vi "Vicon2JointAngles.vi"(5 "Thigh Reference (to Hip)":enum16{"Hip", "Ground"}(ring), 6 "Operation(GetData)":T1, 7 "JointAngleDir([-1,1,1,-1])":dbl[](array[numeric])=[-1.0, 1.0, 1.0, -1.0], 8 "error in (no error)":errorcluster, 9 "LockHipAbduction(F)":bool, 10 "LockHipRotation(T)":bool=TRUE, 11 "ViconIMU in (rad)":dbl[](array[numeric])) -> (0 "error out":errorcluster, 3 "Joint Angles (rad)":dbl[](array[numeric]) format="%#.4f")   [LabVIEW 2016]
uses:
  <vilib>/Analysis/Matrix/Datatypes/RealMatrix.ctl
  HighLevelController/TypeDef/IMU_operation.ctl
  <vilib>/Analysis/coordinate.llb/Euler Rotation Order.ctl
  <vilib>/Analysis/BLAS.llb/LV_Transpose.ctl
  Classes/SerialChain/TypeDef/xyzO.ctl
  <vilib>/Analysis/Matrix/Numeric/Conversions/Array To Matrix - RA2.vi
  <vilib>/Analysis/BLAS.llb/dgemm - General Matrix-Matrix Product (DBL).vi
  <vilib>/Analysis/7linalg.llb/Create Special Real Matrix.vi
  <vilib>/Analysis/NI_AALPro.lvlib
  <vilib>/Analysis/NI_AALBLAS.lvlib
  <vilib>/Analysis/Matrix/NI_Matrix.lvlib
  Classes/SerialChain/SerialChain.lvclass
panel:
  out "R_CtoS_Shank":T2 format="%#.3f"
  out "R_CtoS_Thigh":T2 format="%#.3f"
  out "R_CtoS_Hip":T2 format="%#.3f"
  out "R0":T2 format="%#.3f"
  in  "UseStandPos(T)":bool=TRUE
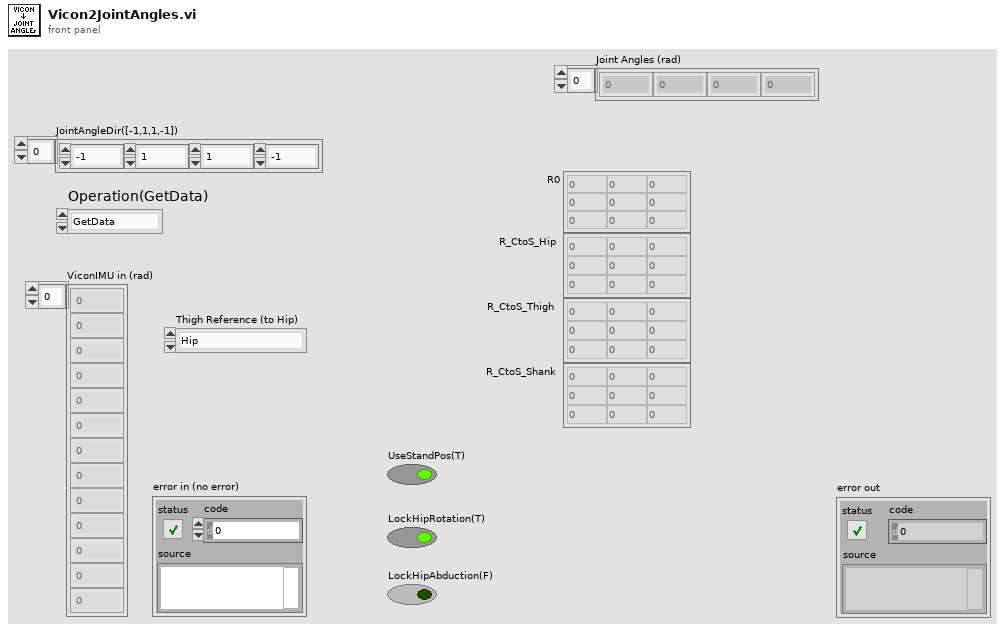
[diagram p1: front panel]
types:
  T1 = typedef "IMU_operation.ctl" = enum16{"GetData", "ClearStandPos", "SetStandPos"}
  T2 = typedef "NI_Matrix.lvlib/RealMatrix.ctl" = dbl[][]
  T3 = typedef "SerialChain.lvclass/xyzO.ctl" = enum16{"X", "Y", "Z", "O"}
  T4 = typedef "NI_AALPro.lvlib/Euler Rotation Order.ctl" = u16
  T5 = typedef "NI_AALBLAS.lvlib/LV_Transpose.ctl" = i32
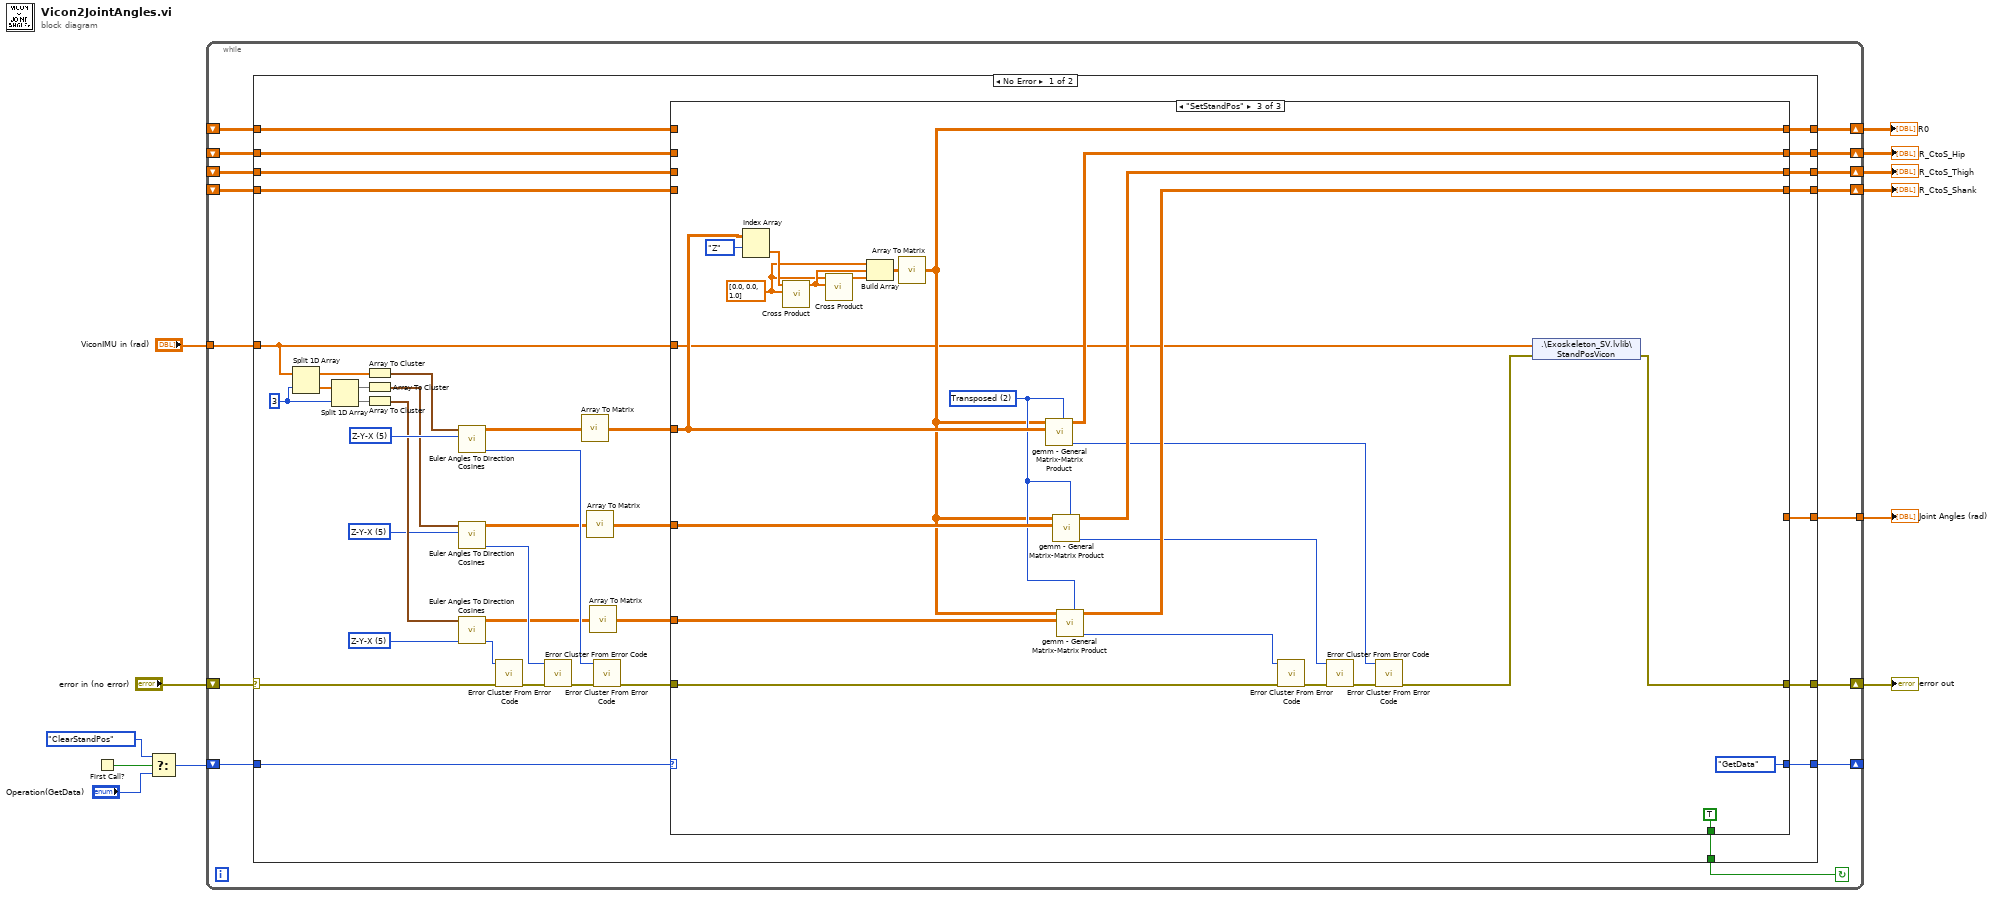
[diagram p0: block diagram]
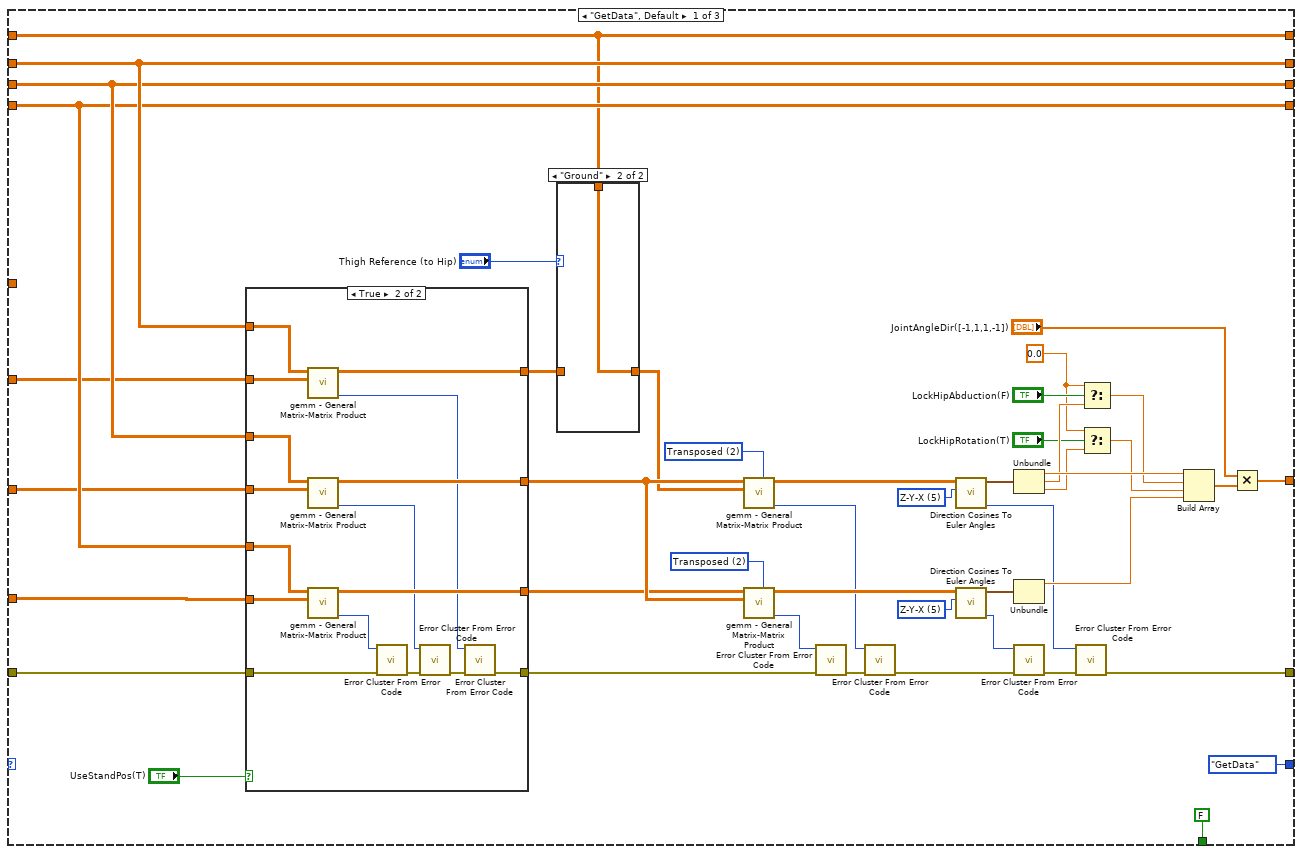
[diagram p2: hidden frame]
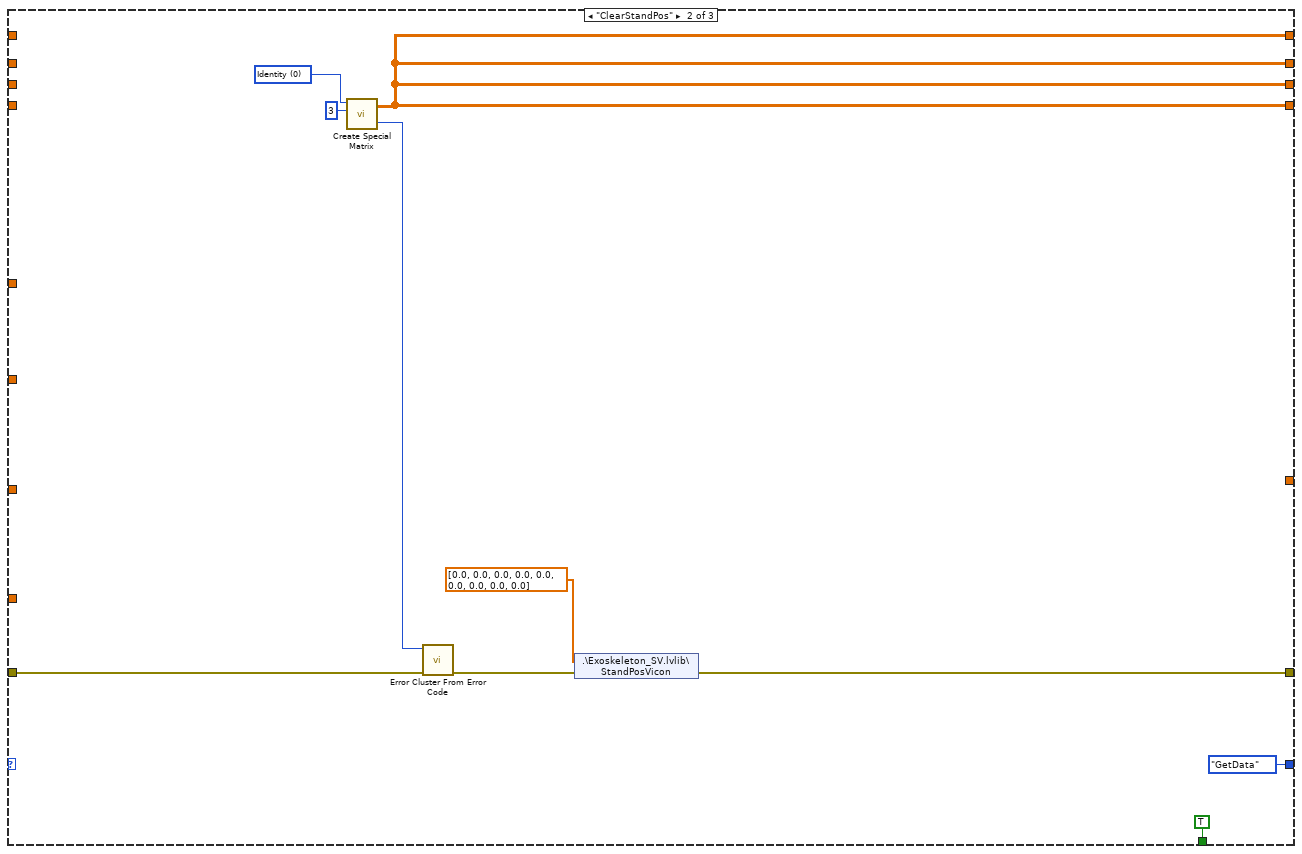
[diagram p5: hidden frame]
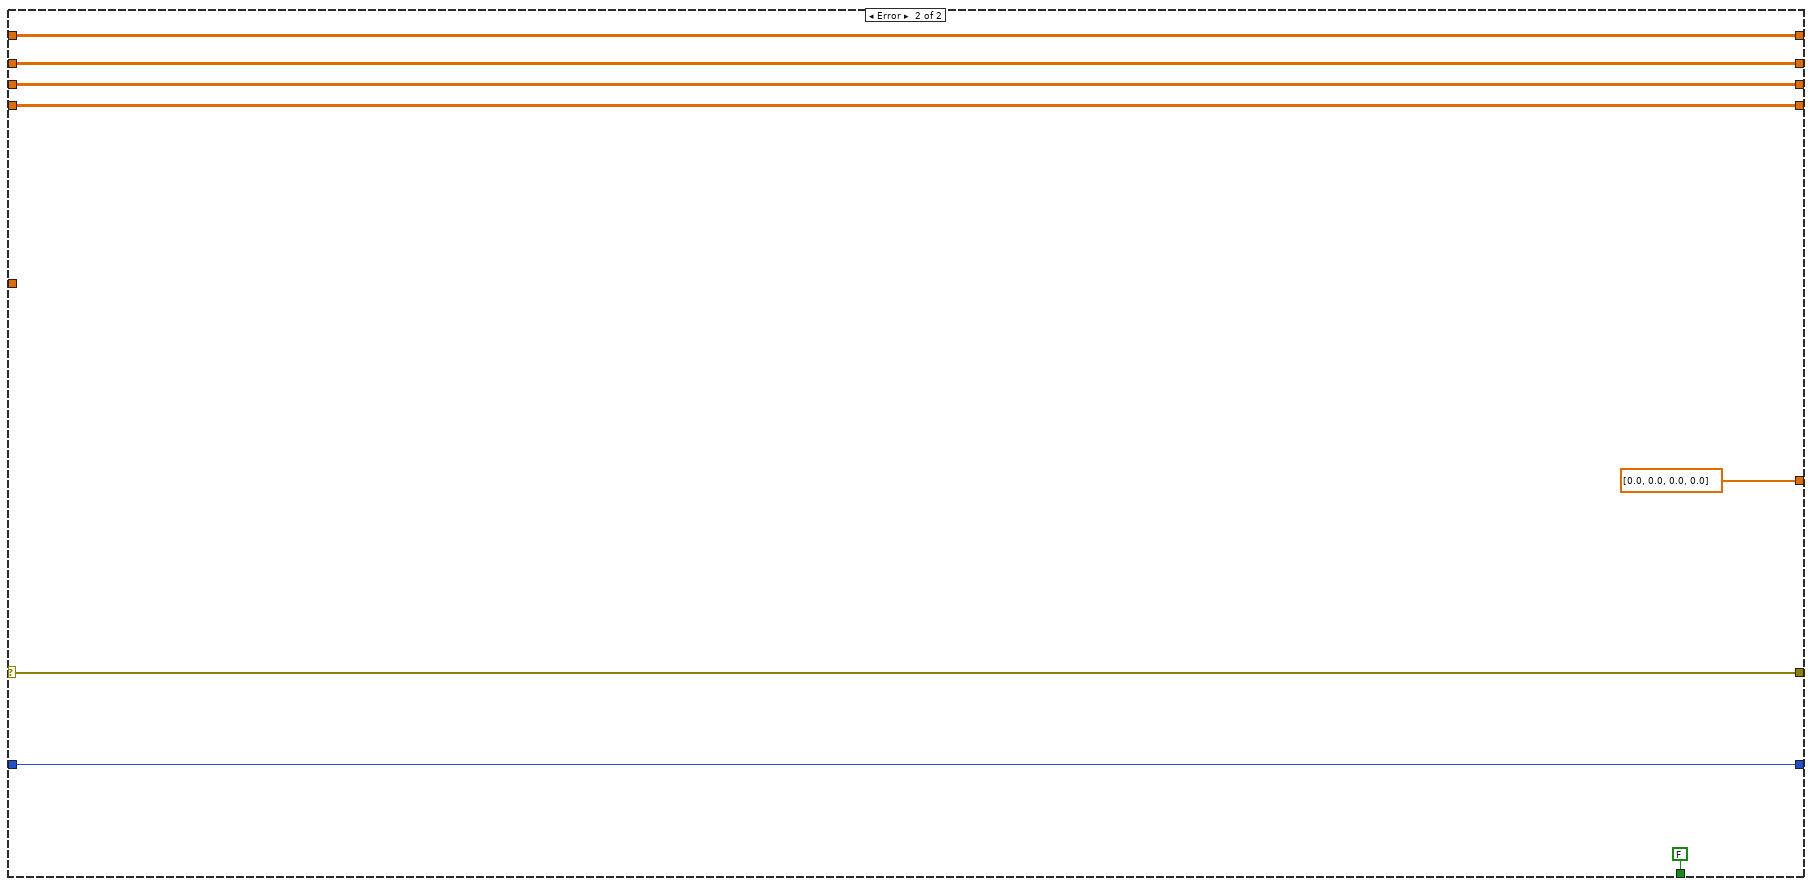
[diagram p6: hidden frame]
diagram:
  n1 = First Call?() -> (First Call?: T/F=w2:bool)
  n2 = Select(t=IMU_operation."ClearStandPos", s=w2, f="Operation(GetData)") -> (s? t:f=w4:T1)
  n3 = while {
    tunnel: [w26] -> w10
    shift-right: [w27] -> w11
    shift-left: "error in (no error)" -> [w25]
    tunnel: "ViconIMU in (rad)" -> [w24]
    shift-right: [w23] -> w8
    shift-left: _ -> [w20]
    shift-right: [w22] -> w7
    shift-left: _ -> [w19]
    shift-right: [w21] -> w6
    shift-left: _ -> [w18]
    shift-right: [w14] -> _
    shift-left: w4 -> [w17]
    shift-right: [w16] -> w5
    shift-left: _ -> [w15]
    stop <- w13 continue-if-true
    n4 = case shown="No Error" w25 {
      selector: w25 -> [w33 w175]
      tunnel: [w65 w175] -> w27
      tunnel: [w64 dbl[] [0.0, 0.0, 0.0, 0.0]] -> w26
      tunnel: w24 -> [w30 _]
      tunnel: [w63 w170] -> w23
      tunnel: [w62 w169] -> w22
      tunnel: [w61 w168] -> w21
      tunnel: w20 -> [w60 w170]
      tunnel: w19 -> [w59 w169]
      tunnel: w18 -> [w58 w168]
      tunnel: w17 -> [w34 w174]
      tunnel: [w32 w171] -> w16
      tunnel: w15 -> [w31 w171]
      tunnel: [w29 w174] -> w14
      tunnel: [w28 FALSE] -> w13
      frame No Error {
        w53 = 3 ("index")
        w44 = T4 5 items=["X-Y-Z", "X-Z-Y", "Y-X-Z", "Y-Z-X", "Z-X-Y", "Z-Y-X", "X-Y-X", "X-Z-X", "Y-X-Y", "Y-Z-Y", "Z-X-Z", "Z-Y-Z"] ("rotation order")
        w41 = T4 5 items=["X-Y-Z", "X-Z-Y", "Y-X-Z", "Y-Z-X", "Z-X-Y", "Z-Y-X", "X-Y-X", "X-Z-X", "Y-X-Y", "Y-Z-Y", "Z-X-Z", "Z-Y-Z"] ("rotation order")
        w39 = T4 5 items=["X-Y-Z", "X-Z-Y", "Y-X-Z", "Y-Z-X", "Z-X-Y", "Z-Y-X", "X-Y-X", "X-Z-X", "Y-X-Y", "Y-Z-Y", "Z-X-Z", "Z-Y-Z"] ("rotation order")
        n5 = Split 1D Array(array=w30, index=w53) -> (first subarray=w56:dbl[], second subarray=w52:dbl[])
        n6 = Split 1D Array(array=w52, index=w53) -> (first subarray=w55:dbl[], second subarray=w54:dbl[])
        n7 = Array To Cluster(array=w56) -> (cluster=w43:cluster{"[0]":dbl, "[1]":dbl, "[2]":dbl})
        n8 = Array To Cluster(array=w55) -> (cluster=w40:cluster{"[0]":dbl, "[1]":dbl, "[2]":dbl})
        n9 = Array To Cluster(array=w54) -> (cluster=w42:cluster{"[0]":dbl, "[1]":dbl, "[2]":dbl})
        n10 = call <vilib>:"Euler Angles To Direction Cosines.vi"("rotation order"=w44, "Euler Angles"=w43) -> ("error"=w57:i32, "Direction Cosines"=w47:dbl[][])  [unwired: 8 in]
        n11 = call <vilib>:"Euler Angles To Direction Cosines.vi"("rotation order"=w39, "Euler Angles"=w40) -> ("error"=w50:i32, "Direction Cosines"=w46:dbl[][])  [unwired: 8 in]
        n12 = call <vilib>:"Euler Angles To Direction Cosines.vi"("rotation order"=w41, "Euler Angles"=w42) -> ("error"=w51:i32, "Direction Cosines"=w45:dbl[][])  [unwired: 8 in]
        n13 = call <vilib>:"Error Cluster From Error Code.vi"("error in (no error)"=w33, "error code (0)"=w51) -> ("error out"=w48:errorcluster)  [unwired: 7 in]
        n14 = call <vilib>:"Error Cluster From Error Code.vi"("error in (no error)"=w48, "error code (0)"=w50) -> ("error out"=w49:errorcluster)  [unwired: 7 in]
        n15 = call-poly <vilib>:"Array To Matrix.vi"("Real 2D Array"=w47) -> ("Real Matrix"=w35:T2)
        n16 = call-poly <vilib>:"Array To Matrix.vi"("Real 2D Array"=w46) -> ("Real Matrix"=w36:T2)
        n17 = call-poly <vilib>:"Array To Matrix.vi"("Real 2D Array"=w45) -> ("Real Matrix"=w37:T2)
        n18 = call <vilib>:"Error Cluster From Error Code.vi"("error in (no error)"=w49, "error code (0)"=w57) -> ("error out"=w38:errorcluster)  [unwired: 7 in]
        n19 = case shown="\"SetStandPos\"" w34 {
          tunnel: [w96 w136 w145] -> w65
          tunnel: [w95 _ _] -> w64
          tunnel: [w88 w133 w158] -> w63
          tunnel: [w87 w133 w157] -> w62
          tunnel: [w86 w133 w156] -> w61
          tunnel: w60 -> [w88 _ _]
          tunnel: w59 -> [w87 _ _]
          tunnel: w58 -> [w86 _ _]
          tunnel: w38 -> [w85 w138 w149]
          tunnel: w37 -> [w84 _ w160]
          tunnel: w36 -> [w83 _ w161]
          tunnel: w35 -> [w82 _ w159]
          tunnel: [w66 w133 w148] -> w32
          tunnel: w31 -> [w66 _ _]
          tunnel: w30 -> [_ _ w147]
          tunnel: [IMU_operation."GetData" ("Operation(GetData)") IMU_operation."GetData" ("Operation(GetData)") IMU_operation."GetData" ("Operation(GetData)")] -> w29
          tunnel: [FALSE TRUE TRUE] -> w28
          frame "GetData", Default {
            w69 = 0.0 ("t")
            w79 = T4 5 items=["X-Y-Z", "X-Z-Y", "Y-X-Z", "Y-Z-X", "Z-X-Y", "Z-Y-X", "X-Y-X", "X-Z-X", "Y-X-Y", "Y-Z-Y", "Z-X-Z", "Z-Y-Z"] ("rotation order")
            w81 = T4 5 items=["X-Y-Z", "X-Z-Y", "Y-X-Z", "Y-Z-X", "Z-X-Y", "Z-Y-X", "X-Y-X", "X-Z-X", "Y-X-Y", "Y-Z-Y", "Z-X-Z", "Z-Y-Z"] ("rotation order")
            w104 = T5 2 items=["Direct", "Conjugated & Transposed", "Transposed"] ("operation B")
            w103 = T5 2 items=["Direct", "Conjugated & Transposed", "Transposed"] ("operation B")
            n20 = case shown="True" "UseStandPos(T)" {
              tunnel: w82 -> [w116 w117]
              tunnel: [w116 w132] -> w90
              tunnel: [w115 w131] -> w102
              tunnel: w83 -> [w115 w128]
              tunnel: w84 -> [w114 w130]
              tunnel: [w114 w129] -> w101
              tunnel: w88 -> [_ w124]
              tunnel: w87 -> [_ w123]
              tunnel: w86 -> [_ w122]
              tunnel: w85 -> [w113 w121]
              tunnel: [w113 w118] -> w99
              frame False {
              }
              frame True {
                n21 = call-poly <vilib>:"gemm - General Matrix-Matrix Product.vi"("B"=w117, "A"=w124) -> ("error"=w127:i32, "dgemm"=w132:T2)  [unwired: 8 in]
                n22 = call-poly <vilib>:"gemm - General Matrix-Matrix Product.vi"("B"=w128, "A"=w123) -> ("error"=w126:i32, "dgemm"=w131:T2)  [unwired: 8 in]
                n23 = call-poly <vilib>:"gemm - General Matrix-Matrix Product.vi"("B"=w130, "A"=w122) -> ("error"=w125:i32, "dgemm"=w129:T2)  [unwired: 8 in]
                n24 = call <vilib>:"Error Cluster From Error Code.vi"("error in (no error)"=w121, "error code (0)"=w125) -> ("error out"=w120:errorcluster)  [unwired: 7 in]
                n25 = call <vilib>:"Error Cluster From Error Code.vi"("error in (no error)"=w120, "error code (0)"=w126) -> ("error out"=w119:errorcluster)  [unwired: 7 in]
                n26 = call <vilib>:"Error Cluster From Error Code.vi"("error in (no error)"=w119, "error code (0)"=w127) -> ("error out"=w118:errorcluster)  [unwired: 7 in]
              }
            }
            n27 = case shown="\"Ground\"" "Thigh Reference (to Hip)" {
              tunnel: w90 -> [w111 _]
              tunnel: [w111 w112] -> w89
              tunnel: w66 -> [_ w112]
              frame "Hip", Default {
              }
              frame "Ground" {
              }
            }
            n28 = call-poly <vilib>:"gemm - General Matrix-Matrix Product.vi"("operation B"=w104, "B"=w89, "A"=w102) -> ("error"=w98:i32, "dgemm"=w105:T2)  [unwired: 7 in]
            n29 = call-poly <vilib>:"gemm - General Matrix-Matrix Product.vi"("operation B"=w103, "B"=w102, "A"=w101) -> ("error"=w97:i32, "dgemm"=w108:T2)  [unwired: 7 in]
            n30 = call <vilib>:"Error Cluster From Error Code.vi"("error in (no error)"=w99, "error code (0)"=w97) -> ("error out"=w94:errorcluster)  [unwired: 7 in]
            n31 = call <vilib>:"Error Cluster From Error Code.vi"("error in (no error)"=w94, "error code (0)"=w98) -> ("error out"=w93:errorcluster)  [unwired: 7 in]
            n32 = call <vilib>:"Direction Cosines To Euler Angles.vi"("rotation order"=w79, "Direction Cosines"=w105) -> ("error"=w77:i32, "Euler Angles"=w78:cluster{"phi":dbl, "theta":dbl, "psi":dbl})  [unwired: 8 in]
            n33 = call <vilib>:"Direction Cosines To Euler Angles.vi"("rotation order"=w81, "Direction Cosines"=w108) -> ("error"=w76:i32, "Euler Angles"=w80:cluster{"phi":dbl, "theta":dbl, "psi":dbl})  [unwired: 8 in]
            n34 = Unbundle(w78) -> ("phi"=w107:dbl, "theta"=w73:dbl, "psi"=w70:dbl)
            n35 = Unbundle(w80) -> ("phi"=w106:dbl)  [unwired: 2 out]
            n36 = call <vilib>:"Error Cluster From Error Code.vi"("error in (no error)"=w93, "error code (0)"=w76) -> ("error out"=w75:errorcluster)  [unwired: 7 in]
            n37 = call <vilib>:"Error Cluster From Error Code.vi"("error in (no error)"=w75, "error code (0)"=w77) -> ("error out"=w96:errorcluster)  [unwired: 7 in]
            n38 = Select(t=w69, s="LockHipAbduction(F)", f=w73) -> (s? t:f=w92:dbl)
            n39 = Select(t=w69, s="LockHipRotation(T)", f=w70) -> (s? t:f=w71:dbl)
            n40 = Build Array(w107, w92, w71, w106) -> (w110:dbl[])
            n41 = Multiply(x="JointAngleDir([-1,1,1,-1])", y=w110) -> (x*y=w95:dbl[])
          }
          frame "ClearStandPos" {
            w140 = 0 items=["Identity", "Diagonal", "Toeplitz", "Vandermonde", "Companion", "Hankel", "Hadamard", "Wilkinson", "Hilbert", "Inverse Hilbert", "Rosser", "Pascal"] ("matrix type")
            n42 = call-poly <vilib>:"Create Special Matrix.vi"("matrix type"=w140, "matrix size"=3) -> ("Special Matrix"=w133:T2, "error"=w139:i32)  [unwired: 3 in]
            n43 = call <vilib>:"Error Cluster From Error Code.vi"("error in (no error)"=w138, "error code (0)"=w139) -> ("error out"=w137:errorcluster)  [unwired: 7 in]
            n44 = shared-variable ".\\Exoskeleton_SV.lvlib\\StandPosVicon"(dbl[] [0.0, 0.0, 0.0, 0.0, 0.0, 0.0, 0.0, 0.0, 0.0] ("ZeroOrient 2"), error in=w137) -> (error out=w136:errorcluster)
          }
          frame "SetStandPos" {
            w155 = T5 2 items=["Direct", "Conjugated & Transposed", "Transposed"] ("operation B")
            w162 = dbl[] [0.0, 0.0, 1.0]
            n45 = Index Array(array=w159, index (row)=xyzO."Z" ("XYZ")) -> (element=w165:dbl[])  [unwired: 1 in]
            n46 = call <vilib>:"Cross Product.vi"("B Vector"=w162, "A Vector"=w165) -> ("Cross Product"=w164:dbl[])  [unwired: 8 in, 1 out]
            n47 = call <vilib>:"Cross Product.vi"("B Vector"=w164, "A Vector"=w162) -> ("Cross Product"=w163:dbl[])  [unwired: 8 in, 1 out]
            n48 = Build Array(w162, w164, w163) -> (w167:dbl[][])
            n49 = call-poly <vilib>:"Array To Matrix.vi"("Real 2D Array"=w167) -> ("Real Matrix"=w148:T2)
            n50 = call-poly <vilib>:"gemm - General Matrix-Matrix Product.vi"("operation B"=w155, "B"=w159, "A"=w148) -> ("error"=w150:i32, "dgemm"=w158:T2)  [unwired: 7 in]
            n51 = call-poly <vilib>:"gemm - General Matrix-Matrix Product.vi"("operation B"=w155, "B"=w161, "A"=w148) -> ("error"=w151:i32, "dgemm"=w157:T2)  [unwired: 7 in]
            n52 = call-poly <vilib>:"gemm - General Matrix-Matrix Product.vi"("operation B"=w155, "B"=w160, "A"=w148) -> ("error"=w152:i32, "dgemm"=w156:T2)  [unwired: 7 in]
            n53 = call <vilib>:"Error Cluster From Error Code.vi"("error in (no error)"=w149, "error code (0)"=w152) -> ("error out"=w154:errorcluster)  [unwired: 7 in]
            n54 = call <vilib>:"Error Cluster From Error Code.vi"("error in (no error)"=w154, "error code (0)"=w151) -> ("error out"=w153:errorcluster)  [unwired: 7 in]
            n55 = call <vilib>:"Error Cluster From Error Code.vi"("error in (no error)"=w153, "error code (0)"=w150) -> ("error out"=w146:errorcluster)  [unwired: 7 in]
            n56 = shared-variable ".\\Exoskeleton_SV.lvlib\\StandPosVicon"(w147, error in=w146) -> (error out=w145:errorcluster)
          }
        }
      }
      frame Error {
      }
    }
  }
  "Joint Angles (rad)" <- w10
  "error out" <- w11
  "R_CtoS_Shank" <- w6
  "R_CtoS_Hip" <- w8
  "R_CtoS_Thigh" <- w7
  "R0" <- w5
